vi "scanTest.vi"() -> ()   [LabVIEW 2013]
panel:
  in  "Line Style":string(combo)="-"
  in  "Marker Shape":string(combo)="*"
  out "error out":errorcluster
  in  "Lancer Matlab":bool
  out "ListofColors":u32[](array[colorbox])
  in  "Array":i32[](array[numeric])
  out "OS":string
  in  "Polydegree Line Width":i32=2 min=0 max=15 step=1
  in  "PolyDegree":i32=3 min=0 max=69 step=1
  in  "Marker Size":i32=2 min=1 max=15 step=1
  in  "Line Width":i32=1 min=0 max=15 step=1
  in  "Wait":i32=3 min=0 max=15 step=1
  out "Nombre de couleur":i32
  out "Hauteur":i16
  out "Largeur":i16
  out "Image ˆ retravailler":picture
  in  "Selectionner une image *.png":path
  out "Affichage des erreurs":string
  # "ScanTest: panneau de control"
  # "Options du Graphique"
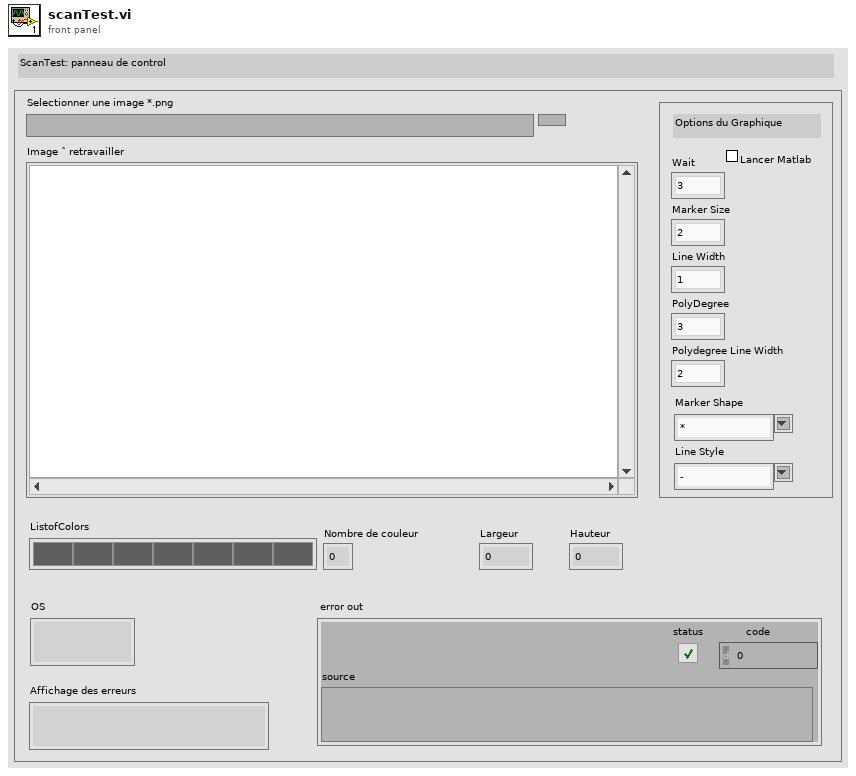
[diagram p1: front panel]
types:
  T1 = enum16{"open", "replace", "create", "open or create", "replace or create", "replace or create with confirmation"}
  T2 = typedef "imagedata.ctl" = cluster{"image type":i32, "image depth":i32, "image":u8[], "mask":u8[], "colors":u32[], "Rectangle":cluster{"left":i16, "top":i16, "right":i16, "bottom":i16}}
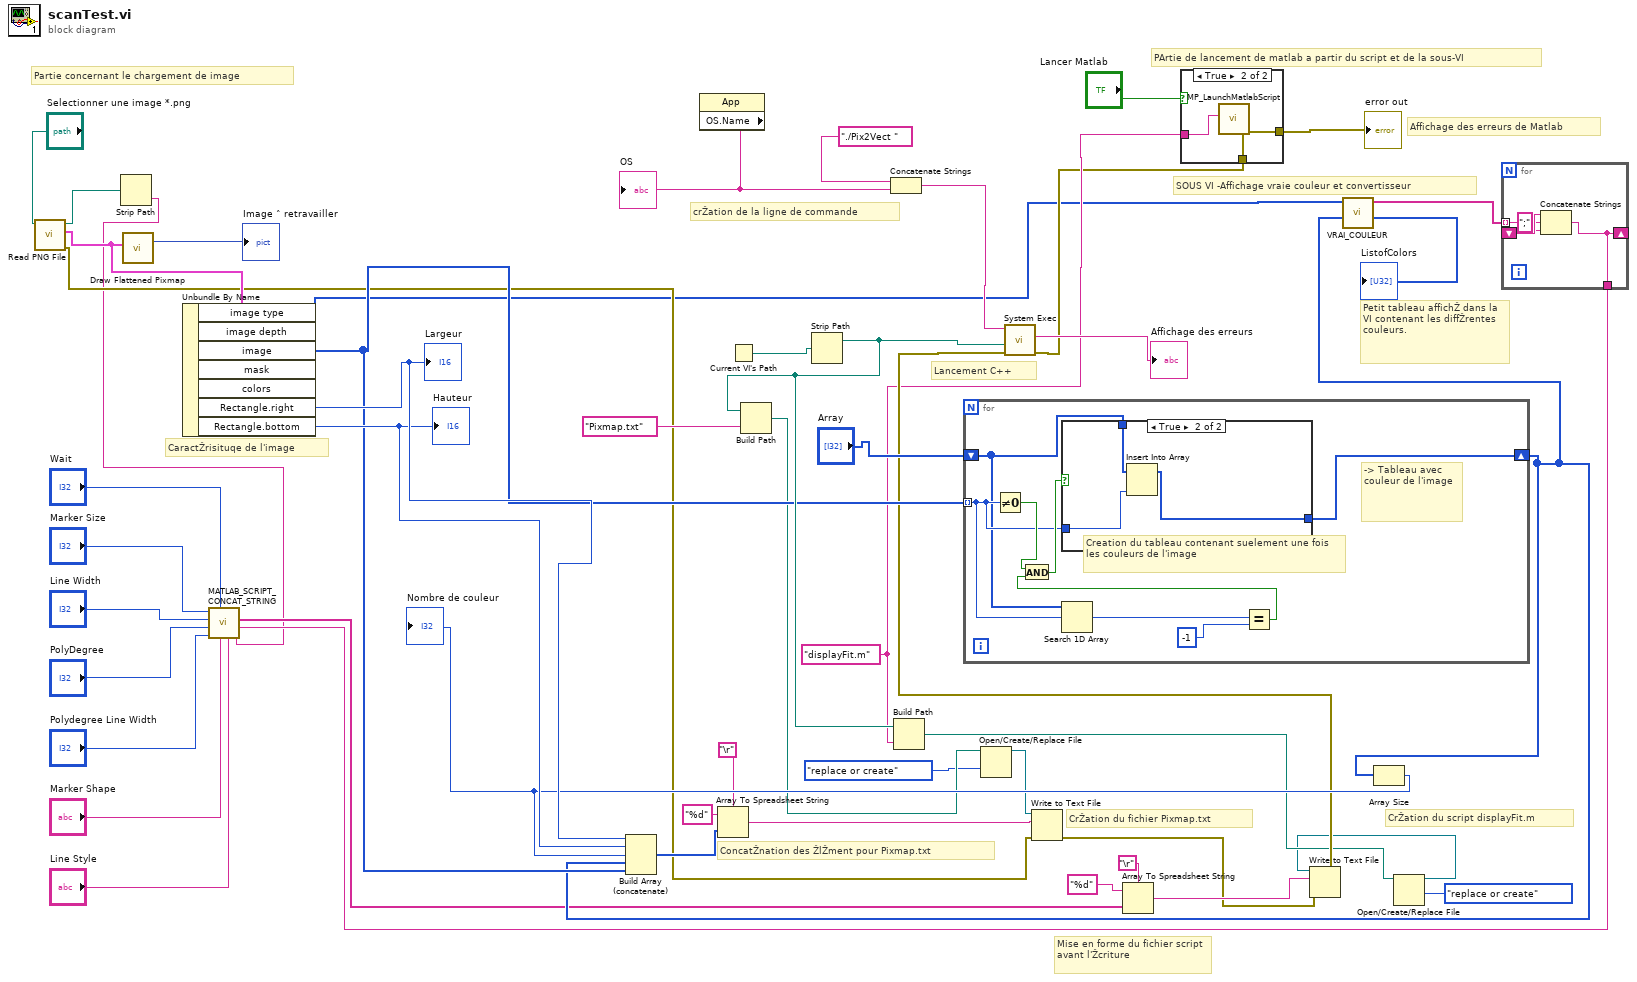
[diagram p0: block diagram]
diagram:
  w20 = "displayFit.m" ("name or relative path")
  # "crŽation de la ligne de commande"
  # "ConcatŽnation des ŽlŽment pour Pixmap.txt"
  # "CrŽation du fichier Pixmap.txt"
  # "Mise en forme du fichier script avant l'Žcriture"
  # "CrŽation du script displayFit.m"
  # "Petit tableau affichŽ dans la VI contenant les diffŽrentes couleurs."
  # "Lancement C++"
  # "Affichage des erreurs de Matlab"
  # "SOUS VI -Affichage vraie couleur et convertisseur"
  # "PArtie de lancement de matlab a partir du script et de la sous-VI"
  # "CaractŽrisituqe de l'image"
  # "Partie concernant le chargement de image"
  n1 = call <vilib>:"Read PNG File.vi"("path to PNG file"="Selectionner une image *.png") -> ("error out"=w29:errorcluster, "image data"=w45:T2, "path"=w33:path)  [unwired: 8 in]
  n2 = Strip Path(path=w33) -> (name=w4:string)  [unwired: 1 out]
  n3 = call <vilib>:"Draw Flattened Pixmap.vi"("image data"=w45) -> ("new picture"=→"Image ˆ retravailler":picture)  [unwired: 8 in]
  n4 = Unbundle By Name(w45) -> ("image"=w31:u8[], "colors"=w15:u32[], "Rectangle.right"=w44:i16, "Rectangle.bottom"=w43:i16)  [unwired: 3 out]
  "Largeur" <- w44
  "Hauteur" <- w43
  n5 = property class="App"() -> ("OS.Name"=w19:string)  [unwired: 2 in, 2 out]
  "OS" <- w19
  n6 = Current VI's Path() -> (path=w49:path)
  n7 = Strip Path(path=w49) -> (stripped path=w34:path)  [unwired: 1 out]
  n8 = Build Path(base path=w34, name or relative path="Pixmap.txt") -> (appended path=w23:path)
  n9 = Concatenate Strings("./Pix2Vect ", w19) -> (w48:string)
  n10 = Build Path(base path=w34, name or relative path=w20) -> (appended path=w25:path)
  n11 = for {
    shift-right: [w55] -> w14
    shift-left: "Array" -> [w54]
    tunnel: w31 -> [w56] mode=indexing
    # "Creation du tableau contenant suelement une fois les couleurs de l'image"
    # "-> Tableau avec couleur de l'image"
    n12 = Not Equal To 0?(x=w56) -> (x != 0?=w58:bool)
    n13 = Search 1D Array(1D array=w54, element=w56) -> (index of element=w53:i32)  [unwired: 1 in]
    n14 = Equal?(x=w53, y=-1) -> (x = y?=w51:bool)
    n15 = And(x=w58, y=w51) -> (x .and. y?=w57:bool)
    n16 = case shown="True" w57 {
      tunnel: w54 -> [w59 w62]
      tunnel: [w59 w61] -> w55
      tunnel: w56 -> [_ w60]
      frame False {
      }
      frame True {
        n17 = Insert Into Array(array=w62, new element=w60) -> (w61:i32[])  [unwired: 1 in]
      }
    }
  }
  n18 = Open/Create/Replace File(file path (use dialog)=w23, operation (0:open)=T1."replace or create") -> (refnum out=w22:refnum<file>)  [unwired: 4 in, 2 out]
  n19 = call "VRAI_COULEUR.vi"("IMAGE COLORS"=w14, "CLUT"=w15) -> ("REAL IMAGE COLORS"=→"ListofColors":i32[], "STRING FOR MATLAB"=w13:string[])  [unwired: 8 in]
  n20 = Array Size(array=w14) -> (size(s)=w41:i32)
  "Nombre de couleur" <- w41
  n21 = Build Array (concatenate)(w44, w43, w41, w14, w31) -> (w42:i32[])
  n22 = Array To Spreadsheet String(delimiter (Tab)="\r", array=w42, 3:"%d" ("format string")) -> (spreadsheet string=w38:string)
  n23 = Write to Text File(file (use dialog)=w22, text=w38, error in=w29) -> (error out=w28:errorcluster)  [unwired: 1 in, 2 out]
  n24 = Open/Create/Replace File(file path (use dialog)=w25, operation (0:open)=T1."replace or create") -> (refnum out=w24:refnum<file>)  [unwired: 4 in, 2 out]
  n25 = for {
    shift-right: [w65] -> _
    shift-left: _ -> [w66]
    tunnel: w13 -> [w64] mode=indexing
    tunnel: [w65] -> w11
    n26 = Concatenate Strings(w66, ";" ("string"), w64) -> (w65:string)
  }
  n27 = call "MATLAB_SCRIPT_CONCAT_STRING.vi"("FILENAME"=w4, "COLOR_STR"=w11, "Line Style"="Line Style", "Marker Shape"="Marker Shape", "Wait"="Wait", "Polydegree Line Width"="Polydegree Line Width", "PolyDegree"="PolyDegree", "Line Width"="Line Width", "Marker Size"="Marker Size") -> ("SCRIPT_STR"=w10:string[])  [unwired: 2 in]
  n28 = Array To Spreadsheet String(delimiter (Tab)="\r", array=w10, 3:"%d" ("format string")) -> (spreadsheet string=w35:string)
  n29 = Write to Text File(file (use dialog)=w24, text=w35, error in=w28) -> (error out=w27:errorcluster)  [unwired: 1 in, 2 out]
  n30 = call <vilib>:"System Exec.vi"("error in (no error)"=w27, "working directory"=w34, "command line"=w48) -> ("error out"=w18:errorcluster, "standard error"=→"Affichage des erreurs":string)  [unwired: 5 in, 2 out]
  n31 = case shown="True" "Lancer Matlab" {
    tunnel: w20 -> [_ w70]
    tunnel: w18 -> [w67 w69]
    tunnel: [w67 w68] -> w17
    frame False {
    }
    frame True {
      n32 = call "MP_LaunchMatlabScript.vi"("error in (no error)"=w69, "matlab script name with extension"=w70) -> ("error out"=w68:errorcluster)  [unwired: 5 in, 4 out]
    }
  }
  "error out" <- w17
